vi "Financial Forecasting.vi"() -> ()   [LabVIEW 2023]
doc: "Forecasts future sales based on the linear fit curve of actual sales. This example displays the actual sales, the linear fit curve of actual sales, and future sales on a graph."
uses:
  <vilib>/Analysis/baseanly.llb/Scale 1D.vi
  <vilib>/Analysis/NI_AALPro.lvlib
  <vilib>/Analysis/NI_AALBase.lvlib
panel:
  out "Forecast Graph":T1(graph)
  out "Forecast Table":string[][](table)
  out "Mean Squared Error":dbl
  in  "Forecast Method":u16(ring) items=["Linear", "Exponential"]
  in  "Sales Data":string[][](table)=[["7/94", "3.377"], ["8/94", "3.185"], ["9/94", "3.560"], ["10/94", "3.623"], ["11/94", "4.102"], ["12/94", "4.304"], ["1/95", "4.083"], ["2/95", "4.064"], ["3/95", "4.639"], ["4/95", "4.020"], ["5/95", "4.153"], ["6/95", "4.425"], ["7/95", "5.838"], ["8/95", "4.167"], ["9/95", "4.332"], ["10/95", "4.642"], ["11/95", "4.308"]]
  # "Overview: Demonstrates the use of the Fitting VIs to calculate forecast data.\nRequirements: LabVIEW Full Development System\nInstructions: \n1. Run the VI.\n2. Change the Forecast Method and run the VI again."
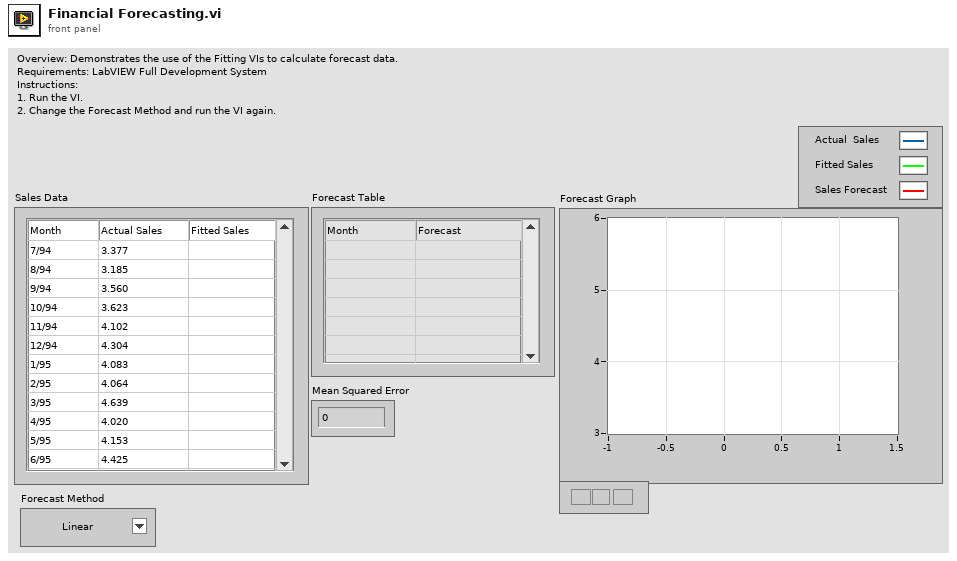
[diagram p1: front panel]
types:
  T1 = cluster{"Y=(X-offset)/scale":dbl[], "Best Exponential Fit":dbl[]}[]
  T2 = cluster{"amp min":dbl, "amp max":dbl, "damping min":dbl, "damping max":dbl, "offset min":dbl, "offset max":dbl}
  T3 = cluster{"Y=(X-offset)/scale":dbl[], "Best Exponential Fit":dbl[]}
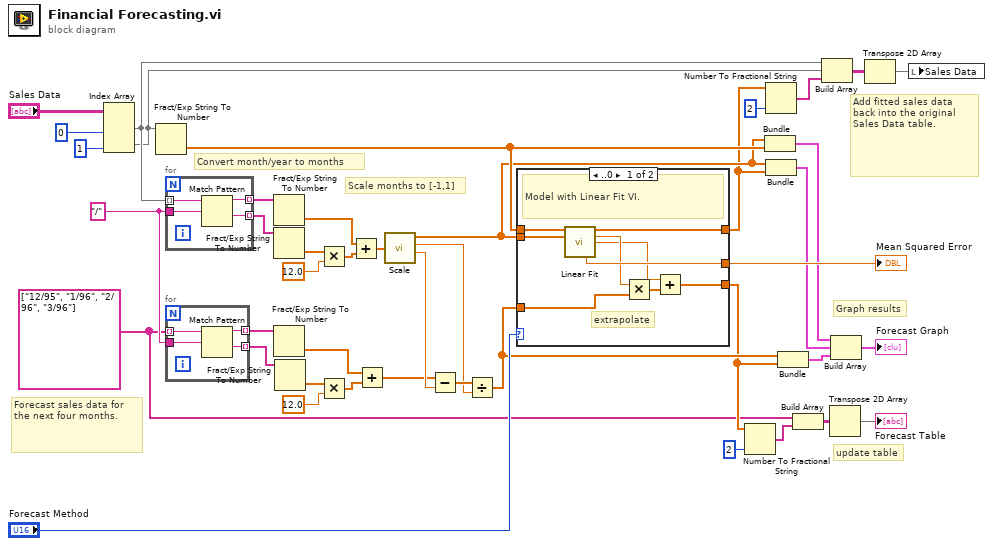
[diagram p0: block diagram]
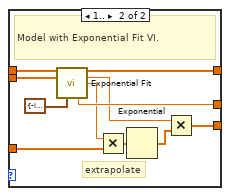
[diagram p2: hidden frame]
diagram:
  w10 = string[] ["12/95", "1/96", "2/96", "3/96"]
  w36 = "/" ("regular expression")
  # "Add fitted sales data back into the original Sales Data table."
  # "Forecast sales data for the next four months."
  # "Convert month/year to months"
  # "Scale months to [-1,1]"
  # "Graph results"
  # "update table"
  n1 = Index Array(array="Sales Data", index (col) #1=0, index (col) #2=1 ("index (col)")) -> (element #1=w6:string[], element #2=w5:string[])  [unwired: 2 in]
  n2 = Fract/Exp String To Number(string=w5) -> (number=w18:dbl[])  [unwired: 3 in, 1 out]
  n3 = for {
    tunnel: w6 -> [w47] mode=indexing
    tunnel: w36 -> [w46]
    tunnel: [w45] -> w40 mode=indexing
    tunnel: [w44] -> w39 mode=indexing
    n4 = Match Pattern(string=w47, regular expression=w46) -> (before substring=w45:string, after substring=w44:string)  [unwired: 1 in, 2 out]
  }
  n5 = for {
    tunnel: w10 -> [w51] mode=indexing
    tunnel: w36 -> [w50]
    tunnel: [w49] -> w33 mode=indexing
    tunnel: [w48] -> w32 mode=indexing
    n6 = Match Pattern(string=w51, regular expression=w50) -> (before substring=w49:string, after substring=w48:string)  [unwired: 1 in, 2 out]
  }
  n7 = Fract/Exp String To Number(string=w40) -> (number=w22:dbl[])  [unwired: 3 in, 1 out]
  n8 = Fract/Exp String To Number(string=w39) -> (number=w21:dbl[])  [unwired: 3 in, 1 out]
  n9 = Fract/Exp String To Number(string=w33) -> (number=w24:dbl[])  [unwired: 3 in, 1 out]
  n10 = Fract/Exp String To Number(string=w32) -> (number=w23:dbl[])  [unwired: 3 in, 1 out]
  n11 = Multiply(x=w21, y=12.0) -> (x*y=w37:dbl[])
  n12 = Multiply(x=w23, y=12.0) -> (x*y=w35:dbl[])
  n13 = Add(x=w22, y=w37) -> (x+y=w20:dbl[])
  n14 = Add(x=w24, y=w35) -> (x+y=w19:dbl[])
  n15 = call-poly <vilib>:"Scale.vi"("X"=w20) -> ("Y=(X-offset)/scale"=w11:dbl[], "scale"=w29:dbl, "offset"=w31:dbl)  [unwired: 1 out]
  n16 = Subtract(x=w19, y=w31) -> (x-y=w30:dbl[])
  n17 = Divide(x=w30, y=w29) -> (x/y=w17:dbl[])
  n18 = case shown="..0" "Forecast Method" {
    tunnel: w11 -> [w60 w70]
    tunnel: w18 -> [w59 w71]
    tunnel: [w58 w62] -> w9
    tunnel: [w57 w69] -> w25
    tunnel: w17 -> [w54 w64]
    tunnel: [w53 w61] -> w16
    frame ..0 {
      # "extrapolate"
      # "Model with Linear Fit VI."
      n19 = call <vilib>:"Linear Fit.vi"("Y"=w59, "X"=w60) -> ("Best Linear Fit"=w58:dbl[], "slope"=w55:dbl, "intercept"=w52:dbl, "residue"=w57:dbl)  [unwired: 9 in, 1 out]
      n20 = Multiply(x=w55, y=w54) -> (x*y=w56:dbl[])
      n21 = Add(x=w52, y=w56) -> (x+y=w53:dbl[])
    }
    frame 1.. {
      # "extrapolate"
      # "Model with Exponential Fit VI."
      n22 = call <vilib>:"Exponential Fit.vi"("Y"=w71, "X"=w70, "parameter bounds"=T2 {"amp min"=-inf, "amp max"=inf, "damping min"=-inf, "damping max"=inf, "offset min"=0.0, "offset max"=0.0}) -> ("Best Exponential Fit"=w62:dbl[], "amplitude"=w63:dbl, "damping"=w65:dbl, "residue"=w69:dbl)  [unwired: 7 in, 2 out]
      n23 = Multiply(x=w65, y=w64) -> (x*y=w66:dbl[])
      n24 = Exponential(1:w66) -> (0:w67:dbl[])
      n25 = Multiply(x=w63, y=w67) -> (x*y=w61:dbl[])
    }
  }
  "Mean Squared Error" <- w25
  n26 = Number To Fractional String(number=w16, precision (6)=i16 2) -> (F-format string=w26:string[])  [unwired: 2 in]
  n27 = Bundle("Y=(X-offset)/scale"=w11, w18) -> (w15:cluster{"Y=(X-offset)/scale":dbl[], dbl[]})  [unwired: 1 in]
  n28 = Number To Fractional String(number=w9, precision (6)=i16 2) -> (F-format string=w4:string[])  [unwired: 2 in]
  n29 = Bundle("Y=(X-offset)/scale"=w11, "Best Exponential Fit"=w9) -> (w14:T3)  [unwired: 1 in]
  n30 = Bundle(w17, w16) -> (w13:cluster{dbl[], dbl[]})  [unwired: 1 in]
  n31 = Build Array(w10, w26) -> (w43:string[][])
  n32 = Build Array(w6, w5, w4) -> (w3:string[][])
  n33 = Transpose 2D Array(2D array=w43) -> (transposed array=→"Forecast Table":string[][])
  n34 = Build Array(w15, w14, w13) -> (→"Forecast Graph":T1)
  n35 = Transpose 2D Array(2D array=w3) -> (transposed array=w2:string[][])
  n36 = local write "Sales Data"(w2) -> ()
